vi "Flush Data to Log File.vi"(8 "error in (no error)":errorcluster, 9 "id ligne":i32, 10 "Data Queue":refnum<queue>, 11 "Logging Configuration":T1) -> (0 "error out":errorcluster)   [LabVIEW 2014, in "PLS Logging.lvlib"]
doc: "Flush the data queue of any pending data and write it to the log file. Close the TDMS file reference."
uses:
  PLS Logging.lvlib
  Logging Configuration.ctl
panel:
  out "backlog size":i32
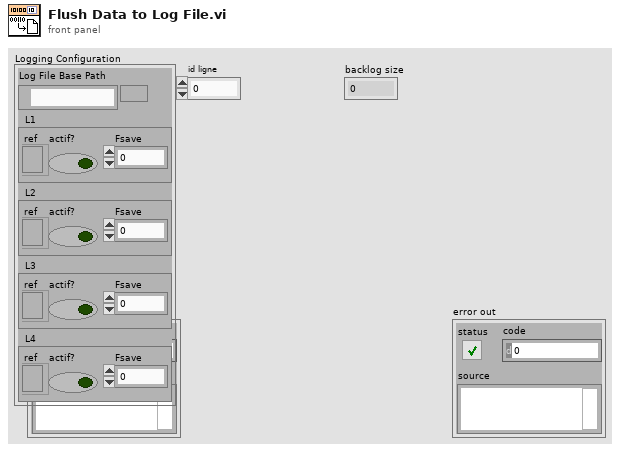
[diagram p1: front panel]
types:
  T1 = typedef "PLS Logging.lvlib/Logging Configuration.ctl" = cluster{"Log File Base Path":path, "L1":cluster{"ref":refnum<file>, "actif?":bool, "Fsave":dbl}, "L2":cluster{"ref":refnum<file>, "actif?":bool, "Fsave":dbl}, "L3":cluster{"ref":refnum<file>, "actif?":bool, "Fsave":dbl}, "L4":cluster{"ref":refnum<file>, "actif?":bool, "Fsave":dbl}}
  T2 = cluster{"ref":refnum<file>, "actif?":bool, "Fsave":dbl}
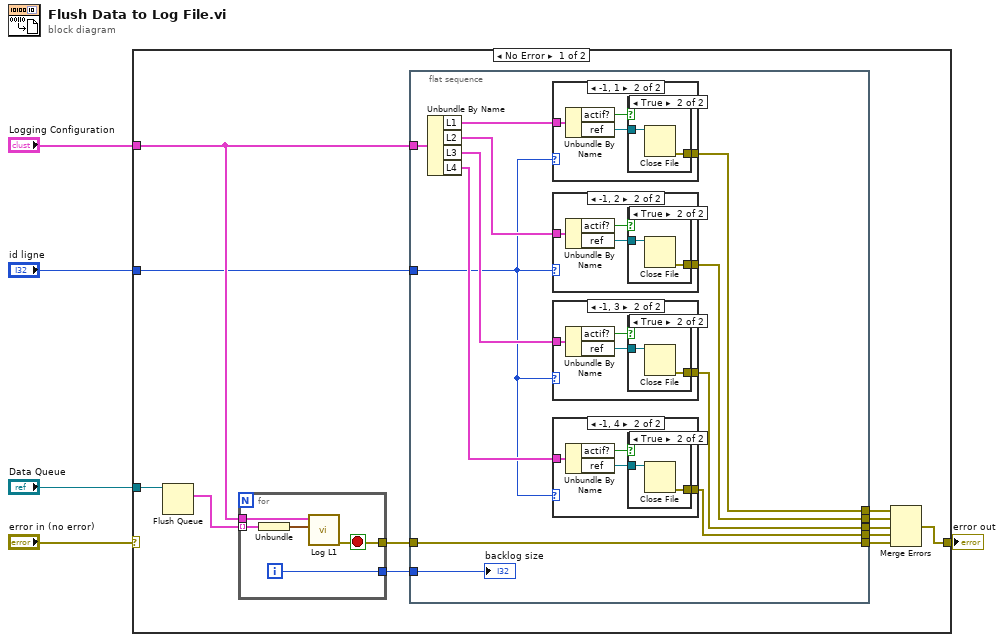
[diagram p0: block diagram]
diagram:
  n1 = case shown="No Error" "error in (no error)" {
    selector: "error in (no error)" -> [_ w59]
    tunnel: "Data Queue" -> [w17 _]
    tunnel: "Logging Configuration" -> [w16 _]
    tunnel: [w13 w59] -> w3
    tunnel: "id ligne" -> [w7 _]
    frame No Error {
      n2 = Flush Queue(queue=w17) -> (remaining elements=w6:cluster{"Array":waveform(dbl)[]}[])  [unwired: 1 in, 2 out]
      n3 = for {
        tunnel: w6 -> [w22] mode=indexing
        tunnel: w16 -> [w20]
        tunnel: [w19] -> w15
        tunnel: [w18] -> w8
        i -> [w18]
        stop <- w19 stop-if-true
        n4 = Unbundle(w22) -> ("Array"=w21:waveform(dbl)[])
        n5 = call "Log L1.vi"("Array"=w21, "Logging Configuration"=w20) -> ("error out"=w19:errorcluster)  [unwired: 9 in]
      }
      n6 = flat-sequence {
        tunnel: w16 -> [w34]
        tunnel: w15 -> [w33]
        tunnel: [w33] -> w14
        tunnel: [w28] -> w12
        tunnel: [w31] -> w11
        tunnel: [w26] -> w10
        tunnel: [w23] -> w9
        tunnel: w8 -> [w30]
        tunnel: w7 -> [w24]
        frame #0 {
          n7 = Unbundle By Name(w34) -> ("L1"=w29:T2, "L2"=w32:T2, "L3"=w27:T2, "L4"=w25:T2)
          n8 = case shown="-1, 1" w24 {
            tunnel: w29 -> [_ w36]
            tunnel: [_ w35] -> w28
            frame Default {
            }
            frame -1, 1 {
              n9 = Unbundle By Name(w36) -> ("actif?"=w38:bool, "ref"=w37:refnum<file>)
              n10 = case shown="True" w38 {
                tunnel: w37 -> [_ w40]
                tunnel: [_ w39] -> w35
                frame False {
                }
                frame True {
                  n11 = Close File(refnum=w40) -> (error out=w39:errorcluster)  [unwired: 1 in, 1 out]
                }
              }
            }
          }
          n12 = case shown="-1, 2" w24 {
            tunnel: w32 -> [_ w54]
            tunnel: [_ w53] -> w31
            frame Default {
            }
            frame -1, 2 {
              n13 = Unbundle By Name(w54) -> ("actif?"=w56:bool, "ref"=w55:refnum<file>)
              n14 = case shown="True" w56 {
                tunnel: w55 -> [_ w58]
                tunnel: [_ w57] -> w53
                frame False {
                }
                frame True {
                  n15 = Close File(refnum=w58) -> (error out=w57:errorcluster)  [unwired: 1 in, 1 out]
                }
              }
            }
          }
          n16 = case shown="-1, 3" w24 {
            tunnel: w27 -> [_ w48]
            tunnel: [_ w47] -> w26
            frame Default {
            }
            frame -1, 3 {
              n17 = Unbundle By Name(w48) -> ("actif?"=w50:bool, "ref"=w49:refnum<file>)
              n18 = case shown="True" w50 {
                tunnel: w49 -> [_ w52]
                tunnel: [_ w51] -> w47
                frame False {
                }
                frame True {
                  n19 = Close File(refnum=w52) -> (error out=w51:errorcluster)  [unwired: 1 in, 1 out]
                }
              }
            }
          }
          n20 = case shown="-1, 4" w24 {
            tunnel: w25 -> [_ w42]
            tunnel: [_ w41] -> w23
            frame Default {
            }
            frame -1, 4 {
              n21 = Unbundle By Name(w42) -> ("actif?"=w44:bool, "ref"=w43:refnum<file>)
              n22 = case shown="True" w44 {
                tunnel: w43 -> [_ w46]
                tunnel: [_ w45] -> w41
                frame False {
                }
                frame True {
                  n23 = Close File(refnum=w46) -> (error out=w45:errorcluster)  [unwired: 1 in, 1 out]
                }
              }
            }
          }
          "backlog size" <- w30
        }
      }
      n24 = Merge Errors(w12, w11, w10, w9, w14) -> (w13:errorcluster)
    }
    frame Error {
    }
  }
  "error out" <- w3
